vi "ImageTest.vi"() -> ()   [LabVIEW 2009]
uses:
  <vilib>/Robotics Library/NIFPGAInterface/DIO/PWMChannel.ctl
  <vilib>/addons/control/pid/pid.llb/PID Control Input Filter (DBL).vi
  <vilib>/Robotics Library/WPI/Camera/Camera.lvlib
  <vilib>/Robotics Library/WPI/PWM/Servo/Servo.lvlib
  <vilib>/addons/control/pid/NI_PID_pid.lvlib
  <vilib>/Robotics Library/WPI/PWM/PWM.lvlib
  <vilib>/Robotics Library/NIFPGAInterface/DIO/NIFPGA DIO.lvlib
panel:
  in  "stop 2":bool
  in  "stop":bool
  out "output":dbl
  in  "Loop Sleep 2":u32=20
  in  "Loop Sleep":u32=20
  in  "Servo Positions":cluster{"X":dbl, "Y":dbl}={"X"=85.52840986947938, "Y"=85.0} {"Y" scale=0.0..170.0; "X" scale=0.0..170.0}
  in  "Smooth":bool=TRUE
  in  "Y Channel":T1=enum."PWM 2"
  in  "X Channel":T1
  out "Image":T2(plugin-control)
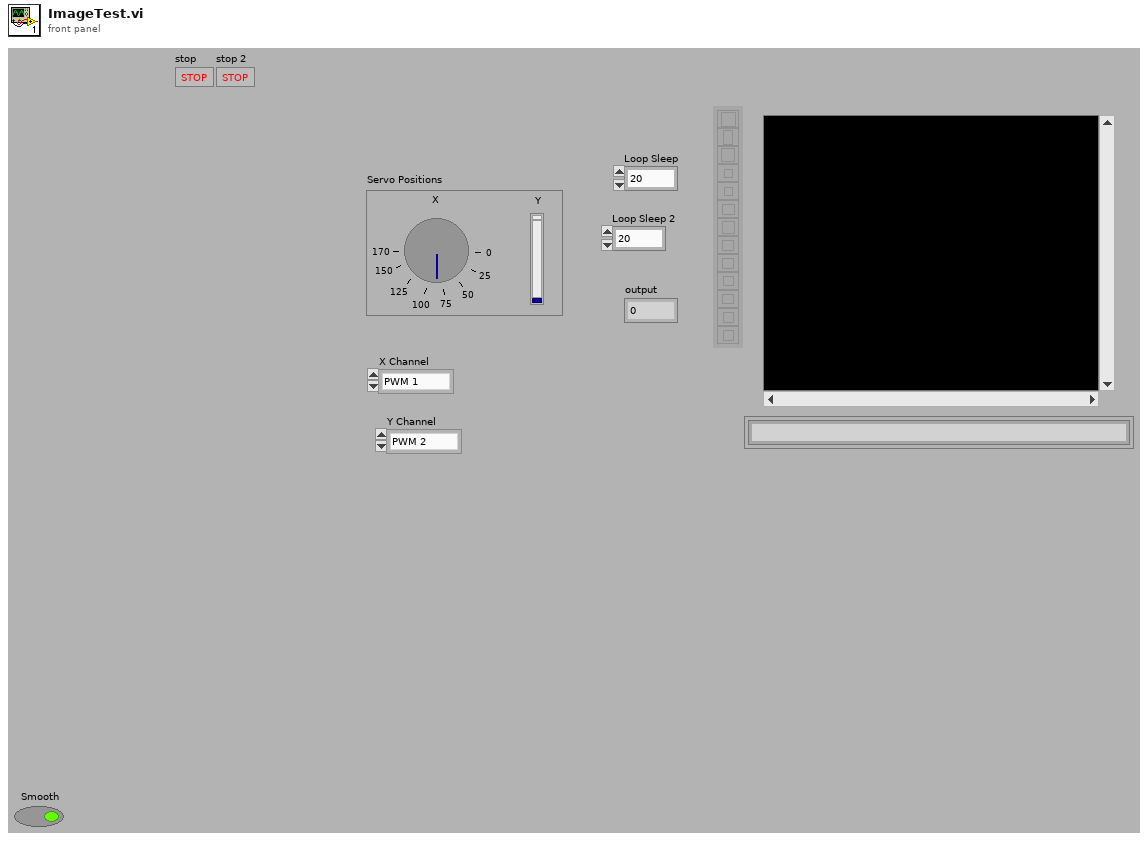
[diagram p1: front panel]
types:
  T1 = typedef "NI_FPGA_Interface.lvlib/NIFPGA DIO.lvlib/PWMChannel.ctl" = enum8{"PWM 1", "PWM 2", "PWM 3", "PWM 4", "PWM 5", "PWM 6", "PWM 7", "PWM 8", "PWM 9", "PWM 10", "Invalid"}
  T2 = typedef "IMAQ Image.ctl" = refnum<image>
  T3 = typedef "Image Type" = u32
  T4 = typedef "Camera.lvlib/CameraDevRef.ctl" = cluster{"Camera Address":string, "CameraStatus":errorcluster, "Session ID":T5}
  T5 = typedef "Camera.lvlib/SessionID.ctl" = i32
  T6 = typedef "PWM.lvlib/PWMDeviceRef.ctl" = cluster{"DeviceStatus":errorcluster, "DIO Module":T7, "PWM Channel":T1, "Invert":bool, "TransformRef":T8, "InvTransformRef":T8, "DeadBand":T9}
  T7 = typedef "NI_FPGA_Interface.lvlib/DigitalModule.ctl" = enum16{"Default", "Slot 4", "Slot 6"}
  T8 = typedef "PWM.lvlib/Transform_ConPane.ctl" = refnum<vi>
  T9 = typedef "PWM.lvlib/Deadband.ctl" = cluster{"Name":string, "maxPositivePwm":i32, "minPositivePwm":i32, "centerPwm":i32, "maxNegativePwm":i32, "minNegativePwm":i32, "angularRange":u16}
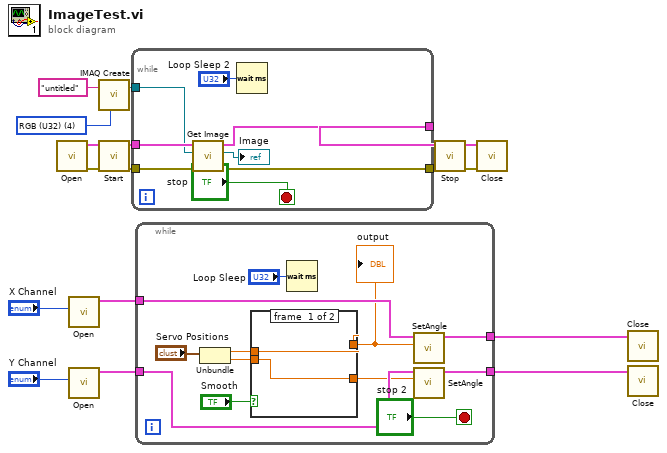
[diagram p0: block diagram]
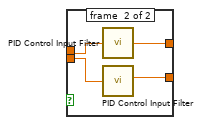
[diagram p2: hidden frame]
diagram:
  w11 = T3 4 items=["Grayscale (U8)", "Grayscale (I16)", "Grayscale (SGL)", "Complex (CSG)", "RGB (U32)", "HSL (U32)", "RGB (U64)", "Grayscale (U16)"] ("Image Type")
  n1 = call <vilib>:"Open.vi"() -> ("error out"=w16:errorcluster, "CameraDevRef"=w17:T4)  [unwired: 10 in]
  n2 = call <vilib>:"Open.vi"("PWM Channel"="X Channel") -> ("PWMDeviceRef"=w4:T6)  [unwired: 9 in, 1 out]
  n3 = call <vilib>:"Open.vi"("PWM Channel"="Y Channel") -> ("PWMDeviceRef"=w2:T6)  [unwired: 9 in, 1 out]
  n4 = call "IMAQ Create"("Image Name"="untitled", "Image Type"=w11) -> ("New Image"=w13:T2)  [unwired: 3 in, 1 out]
  n5 = call <vilib>:"Start.vi"("error in (no error)"=w16, "CameraDevRef"=w17) -> ("error out"=w14:errorcluster, "CameraDevRef Out"=w15:T4)  [unwired: 8 in]
  n6 = while {
    tunnel: w15 -> [w25]
    tunnel: w14 -> [w24]
    tunnel: [w22] -> w10
    tunnel: [w21] -> w9
    tunnel: w13 -> [w23]
    stop <- "stop" stop-if-true
    n7 = call <vilib>:"Get Image.vi"("error in (no error)"=w24, "Image"=w23, "CameraDevRef"=w25) -> ("error out"=w21:errorcluster, "Image Out"=→"Image":T2, "CameraDevRef Out"=w22:T4)  [unwired: 6 in]
    n8 = Wait (ms)(milliseconds to wait="Loop Sleep 2") -> ()  [unwired: 1 out]
  }
  n9 = while {
    tunnel: w4 -> [w35]
    tunnel: [w37] -> w3
    tunnel: w2 -> [w34]
    tunnel: [w33] -> w1
    stop <- "stop 2" stop-if-true
    n10 = Unbundle("Servo Positions") -> ("X"=w31:dbl, "Y"=w29:dbl)
    n11 = case shown="True" "Smooth" {
      tunnel: w31 -> [w39 w43]
      tunnel: [w39 w42] -> w30
      tunnel: w29 -> [w38 w41]
      tunnel: [w38 w40] -> w28
      frame #0 {
      }
      frame #1 {
        n12 = call-poly <vilib>:"PID Control Input Filter.vi"("input"=w43) -> ("output"=w42:dbl)  [unwired: 4 in]
        n13 = call-poly <vilib>:"PID Control Input Filter.vi"("input"=w41) -> ("output"=w40:dbl)  [unwired: 4 in]
      }
    }
    "output" <- w30
    n14 = Wait (ms)(milliseconds to wait="Loop Sleep") -> ()  [unwired: 1 out]
    n15 = call <vilib>:"SetAngle.vi"("Angle"=w30, "PWMDeviceRef"=w35) -> ("PWMDeviceRef"=w37:T6)  [unwired: 8 in, 1 out]
    n16 = call <vilib>:"SetAngle.vi"("Angle"=w28, "PWMDeviceRef"=w34) -> ("PWMDeviceRef"=w33:T6)  [unwired: 8 in, 1 out]
  }
  n17 = call <vilib>:"Stop.vi"("error in (no error)"=w9, "CameraDevRef"=w10) -> ("error out"=w8:errorcluster, "CameraDevRef Out"=w7:T4)  [unwired: 8 in]
  n18 = call <vilib>:"Close.vi"("error in (no error)"=w8, "CameraDevRef"=w7) -> ()  [unwired: 9 in, 1 out]
  n19 = call <vilib>:"Close.vi"("PWMDeviceRef"=w3) -> ()  [unwired: 10 in, 1 out]
  n20 = call <vilib>:"Close.vi"("PWMDeviceRef"=w1) -> ()  [unwired: 10 in, 1 out]
